vi "Deserialise content.vi"(8 "error in (no error)":errorcluster, 10 "JSON String to decode":string, 11 "object in":refnum<class "execute_result Message.lvclass">) -> (0 "error out":errorcluster, 3 "object out":refnum<class "execute_result Message.lvclass">)   [LabVIEW 2018, in "ClientMessaging.lvlib" / "execute_result Message.lvclass"]
uses:
  execute_result Message.lvclass
  C:/Users/gavin/Documents/LabVIEW Data/LabVIEW-Bits/Connectivity/Jupyter Client/IOPub Messages/display_data Message/display_data Message.lvclass
  0d980ed6-cbe1-4885-aae6-970a35042a53.vi
  0a5f0c6c-0550-4779-96c0-91d399c5f344.vi
  0d980ed6-cbe1-4885-aae6-970a35042a53.vi/1a3d486d-82ac-428c-95b3-0a9ad05cfe5a.vi
  0d980ed6-cbe1-4885-aae6-970a35042a53.vi/ef285cc2-6e0a-456a-857a-12896048efb9.vi
  0d980ed6-cbe1-4885-aae6-970a35042a53.vi/c6398968-d40a-4a3c-b292-f485dc4e870e.vi
  0a5f0c6c-0550-4779-96c0-91d399c5f344.vi/34b17207-db4e-493b-b420-69008f9f2caa.vi
  0a5f0c6c-0550-4779-96c0-91d399c5f344.vi/3b460819-9a07-4a15-b3f7-315822020f9d.vi
  0a5f0c6c-0550-4779-96c0-91d399c5f344.vi/19bafac1-6471-4fc4-aca3-faaf461c3460.vi
  <vilib>/JDP Science/JSONtext/Find Item.vi
  <vilib>/JDP Science/JSONtext/String Subset.vi
  <vilib>/JDP Science/JSONtext/Parsing/Parse Full Path or Item Name.vi
  <vilib>/JDP Science/JSONtext/Offset/Find Item Locations by Path.vi
  <vilib>/JDP Science/JSONtext/JSON text to Variant.vi
  Utility/Join Strings in node-path.vi
  Base Classes/Message Class/Message Class.lvclass
  display_data Message/display_data Message.lvclass
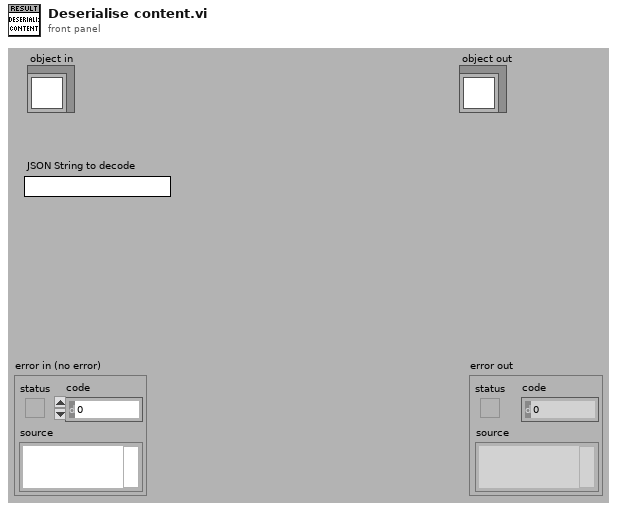
[diagram p1: front panel]
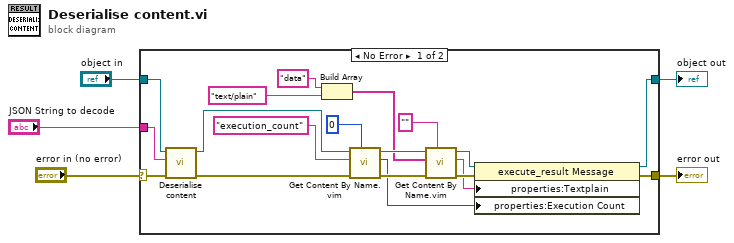
[diagram p0: block diagram]
diagram:
  n1 = case shown="No Error" "error in (no error)" {
    selector: "error in (no error)" -> [w22 w26]
    tunnel: [w8 w26] -> w4
    tunnel: [w10 w25] -> w2
    tunnel: "object in" -> [w24 w25]
    tunnel: "JSON String to decode" -> [w23 _]
    frame No Error {
      n2 = call-parent "Deserialise content.vi"("error in (no error)"=w22, "JSON String to decode"=w23, "object in"=w24) -> ("error out"=w21:errorcluster, "object out"=w20:refnum<class "execute_result Message.lvclass">)  [unwired: 7 in]
      n3 = Build Array("data" ("Name of Content Item"), "text/plain" ("Element Name")) -> (w14:string[])
      n4 = call "Get Content By Name.vim"("Type of content"=0, "error in (no error)"=w21, "Name of Content Item"="execution_count" ("Element Name"), "Message In"=w20) -> ("error out"=w17:errorcluster, "Data Out"=w6:i32, "Message Out"=w16:refnum<class "execute_result Message.lvclass">)  [unwired: 5 in]
      n5 = call "Get Content By Name.vim"("Type of content"="", "error in (no error)"=w17, "Name of Content Item"=w14, "Message In"=w16) -> ("error out"=w9:errorcluster, "Data Out"=w7:string, "Message Out"=w11:refnum<class "execute_result Message.lvclass">)  [unwired: 5 in]
      n6 = property class="execute_result Message"(reference=w11, error in=w9, "properties:Textplain"=w7, "properties:Execution Count"=w6) -> (reference out=w10:refnum<class "execute_result Message.lvclass">, error out=w8:errorcluster)
    }
    frame Error {
    }
  }
  "error out" <- w4
  "object out" <- w2
